vi "Pigeon2 Robot Centric.vi"(10 "Robot Centric Velocities":T1, 11 "PigeonIMUDevRef":T2={"DeviceStatus"={"status"=FALSE, "code"=0, "source"=""}, "Device Number"=0, "Type"=352321536, "Device ID"=0, "Handle"=0, "UsageFrame"=0, "Library Path"=path ""} {"Type" items=["CAN"=352321536, "TalonSRX"=33554432]}) -> (3 "Field Centric Velocities":T1)   [LabVIEW 2023]
uses:
  <vilib>/Rock Robotics/WPI/ThirdParty/Phoenix-LabVIEW/Pigeon IMU/CTRE_PigeonIMU_DeviceRef.ctl
  <vilib>/Rock Robotics/WPI/ThirdParty/Phoenix-LabVIEW/Pigeon IMU/CTRE_PigeonIMU_ConnectionType.ctl
  Type Definitions/Data/Robot Velocities.ctl
  <vilib>/Rock Robotics/WPI/ThirdParty/Phoenix-LabVIEW/Pigeon IMU/CTRE_PigeonIMU_GetYPR.vi
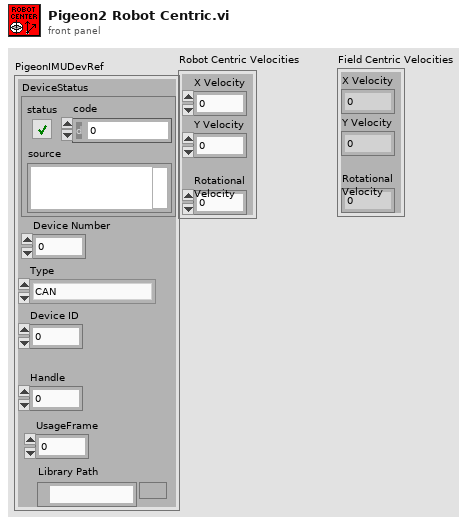
[diagram p1: front panel]
types:
  T1 = typedef "Robot Velocities.ctl" = cluster{"X Velocity":dbl, "Y Velocity":dbl, "Rotational \nVelocity":dbl}
  T2 = typedef "CTRE_PigeonIMU_DeviceRef.ctl" = cluster{"DeviceStatus":errorcluster, "Device Number":u8, "Type":T3, "Device ID":u32, "Handle":u64, "UsageFrame":u32, "Library Path":path}
  T3 = typedef "CTRE_PigeonIMU_ConnectionType.ctl" = u32
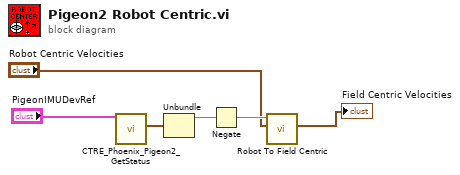
[diagram p0: block diagram]
diagram:
  n1 = call-poly <vilib>:"CTRE_Phoenix_Pigeon2_GetStatus.vi"("PigeonIMUDevRef"="PigeonIMUDevRef") -> ("Yaw Pitch Roll"=w6:cluster{"Yaw":dbl, "Pitch":dbl, "Roll":dbl})  [unwired: 8 in, 2 out]
  n2 = Unbundle(w6) -> ("Yaw"=w5:dbl)  [unwired: 2 out]
  n3 = Negate(x=w5) -> (-x=w3:dbl)
  n4 = call "Robot To Field Centric.vi"("Robot Centric Velocities"="Robot Centric Velocities", "IMU Value (offset)"=w3) -> ("Field Centric Velocities"=→"Field Centric Velocities":T1)  [unwired: 8 in, 1 out]
